vi "Initialize Output Channel Values.vi"(8 "error in (no error)":errorcluster, 11 "Output Process in":refnum<class "Sine Process.lvclass">) -> (0 "error out":errorcluster, 3 "Output Process out":refnum<class "Sine Process.lvclass">)   [LabVIEW 2019, in "TimingDRV Engine.lvlib" / "Sine Process.lvclass"]
uses:
  Sine Process.lvclass
  C:/Users/XEnderMD/Desktop/CD Project Tools/Source/Engine/Windows/Parent Classes/Process/Process.lvclass
  <vilib>/NI VeriStand/Custom Device API/Custom Device Channel Type.ctl
  Parent Classes/Process/Process.lvclass/Process.ctl
  Sine Process.lvclass/Sine Process.ctl
  <vilib>/NI VeriStand/Custom Device API/Custom Device API.lvlib
  Parent Classes/Process/Process.lvclass
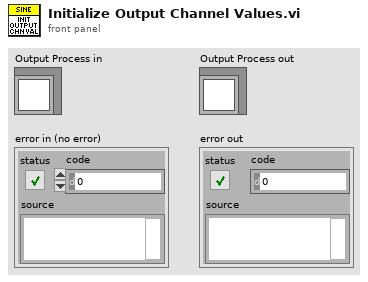
[diagram p1: front panel]
types:
  T1 = typedef "Custom Device API.lvlib/Custom Device Channel Type.ctl" = enum16{"Input", "Output"}
  T2 = typedef "TimingDRV Engine.lvlib/Process.lvclass/Async Paramters.ctl" = cluster{"Device Reference":T3, "Device Clock":string, "Device Inputs FIFO":refnum<k33>, "Device Outputs FIFO":refnum<k33>, "CD Engine Event Ref":T4}
  T3 = typedef "Custom Device API.lvlib/Custom Device Item Ref.ctl" = u64
  T4 = typedef "Custom Device API.lvlib/Custom Device Engine Event Ref.ctl" = refnum<event-registration>
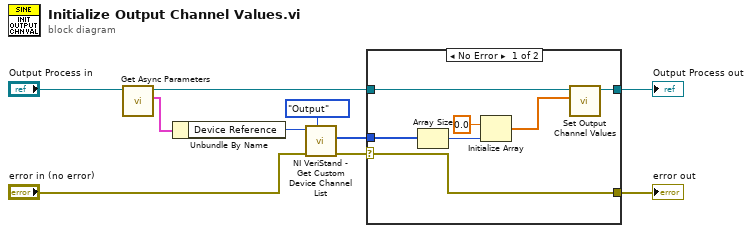
[diagram p0: block diagram]
diagram:
  n1 = call "Get Async Parameters.vi"("Process in"="Output Process in") -> ("Async Parameters"=w3:T2, "Process out"=w1:refnum<class "Sine Process.lvclass">)  [unwired: 9 in]
  n2 = Unbundle By Name(w3) -> ("Device Reference"=w2:T3)
  n3 = call <vilib>:"NI VeriStand - Get Custom Device Channel List.vi"("Channel Type"=Custom_Device_Channel_Type."Output", "error in (no error)"="error in (no error)", "Device Ref in"=w2) -> ("error out"=w8:errorcluster, "Specified Channel Ref List"=w6:T3[])  [unwired: 7 out]
  n4 = case shown="No Error" w8 {
    selector: w8 -> [w13 w18]
    tunnel: w6 -> [w16 _]
    tunnel: w1 -> [w15 w19]
    tunnel: [w13 w18] -> w9
    tunnel: [w12 w19] -> w10
    frame No Error {
      n5 = Array Size(array=w16) -> (size(s)=w11:i32)
      n6 = Initialize Array(0.0 ("element"), w11) -> (w14:dbl[])
      n7 = call "Set Output Channel Values.vi"("Output Channel Values"=w14, "Output Process in"=w15) -> ("Output Process out"=w12:refnum<class "Sine Process.lvclass">)  [unwired: 9 in]
    }
    frame Error {
    }
  }
  "Output Process out" <- w10
  "error out" <- w9
